vi "MatchRegExToSubstringOffsets.vi"(5 "MatchOptions":u32 format="%.0x", 7 "CompileOptions":u32 format="%.0x", 8 "error in":errorcluster, 9 "offset (0)":i32, 10 "search pattern":string, 11 "string":string) -> (0 "error out":errorcluster, 1 "NoMatch?":bool, 2 "OffsetsPastMatch":i32[](array[numeric]), 3 "MatchOffsets":i32[](array[numeric]))   [LabVIEW 2021, in "libpcre2-8.lvlib"]
uses:
  libpcre2-8.lvlib
  Pcre2GetOvectorPointer8.vi
  Pcre2CompileError.vi
  Pcre2ErrorNull.vi
  Pcre2LibError.vi
  Pcre2FnkCallError.vi
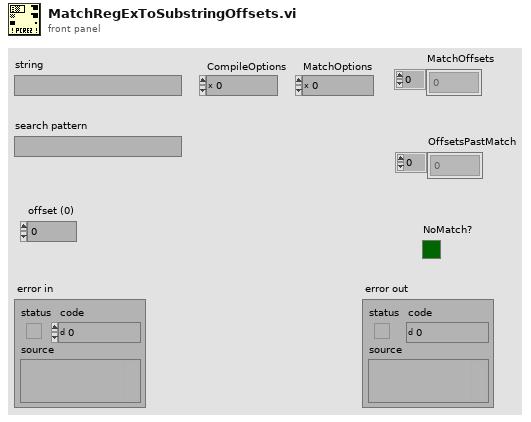
[diagram p1: front panel]
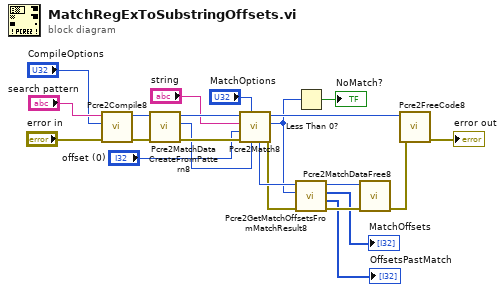
[diagram p0: block diagram]
diagram:
  n1 = call "Pcre2Compile8.vi"("error in"="error in", "Options"="CompileOptions", "Pattern"="search pattern") -> ("error out"=w20:errorcluster, "pCode"=w19:u64)  [unwired: 7 in]
  n2 = call "Pcre2MatchDataCreateFromPattern8.vi"("error in"=w20, "pCode"=w19) -> ("error out"=w21:errorcluster, "pMatchData"=w18:u64, "pCode"=w22:u64)  [unwired: 7 in]
  n3 = call "Pcre2Match8.vi"("pMatchData"=w18, "Options"="MatchOptions", "error in"=w21, "StartOffset"="offset (0)", "Subject"="string", "pCode"=w22) -> ("error out"=w4:errorcluster, "MatchResult"=w3:i32, "pCode"=w17:u64, "pMatchData"=w6:u64)  [unwired: 2 in]
  n4 = Less Than 0?(x=w3) -> (x < 0?=→"NoMatch?":bool)
  n5 = call "Pcre2GetMatchOffsetsFromMatchResult8.vi"("error in"=w4, "MatchResult"=w3, "pMatchData"=w6) -> ("error out"=w12:errorcluster, "OffsetsPastMatch"=→"OffsetsPastMatch":i32[], "MatchOffsets"=→"MatchOffsets":i32[], "pMatchData"=w11:u64)  [unwired: 5 in]
  n6 = call "Pcre2MatchDataFree8.vi"("error in"=w12, "pMatchData"=w11) -> ("error out"=w16:errorcluster)  [unwired: 9 in]
  n7 = call "Pcre2FreeCode8.vi"("error in"=w16, "pCode"=w17) -> ("error out"=→"error out":errorcluster)  [unwired: 9 in]
